vi "Read Chirp.vi"(8 "error in (no error)":errorcluster, 11 "PAS in":refnum<class "PAS.lvclass">) -> (0 "error out":errorcluster, 2 "Chirp":cluster{"f_center":dbl, "bandwidth":dbl}={"f_center"=1350.0, "bandwidth"=150.0}, 3 "PAS out":refnum<class "PAS.lvclass">)   [LabVIEW 2018, in "PAS Library.lvlib" / "PAS.lvclass"]
uses:
  PAS.lvclass
  PAS.lvclass/PAS.ctl
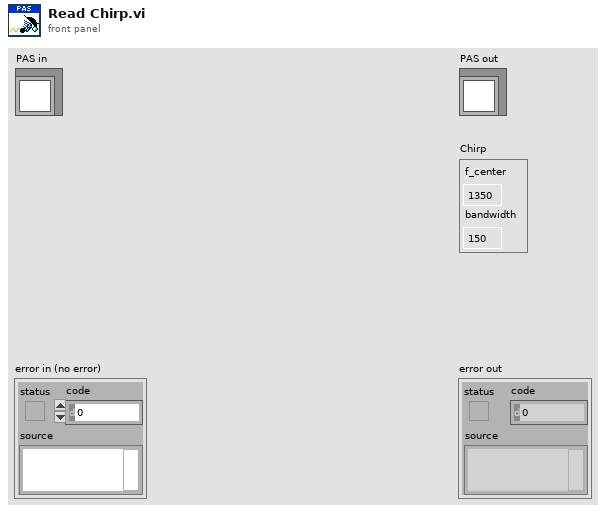
[diagram p1: front panel]
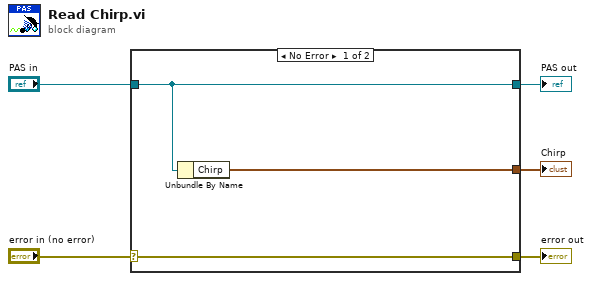
[diagram p0: block diagram]
diagram:
  n1 = case shown="No Error" "error in (no error)" {
    selector: "error in (no error)" -> [w8 w9]
    tunnel: [w8 w9] -> w4
    tunnel: [w7 w10] -> w2
    tunnel: "PAS in" -> [w7 w10]
    tunnel: [w6 _] -> w1
    frame No Error {
      n2 = Unbundle By Name(w7) -> ("Chirp"=w6:cluster{"f_center":dbl, "bandwidth":dbl})
    }
    frame Error {
    }
  }
  "error out" <- w4
  "PAS out" <- w2
  "Chirp" <- w1
